vi "Send SMTP.vi"(5 "Attachment file path name":path, 6 "Body":string, 7 "Subject":string, 8 "error in (no error)":errorcluster, 9 "to":string, 10 "from":string, 11 "mail host":string="mailhost.btw-inc.com") -> (0 "error out":errorcluster)   [LabVIEW 2013]
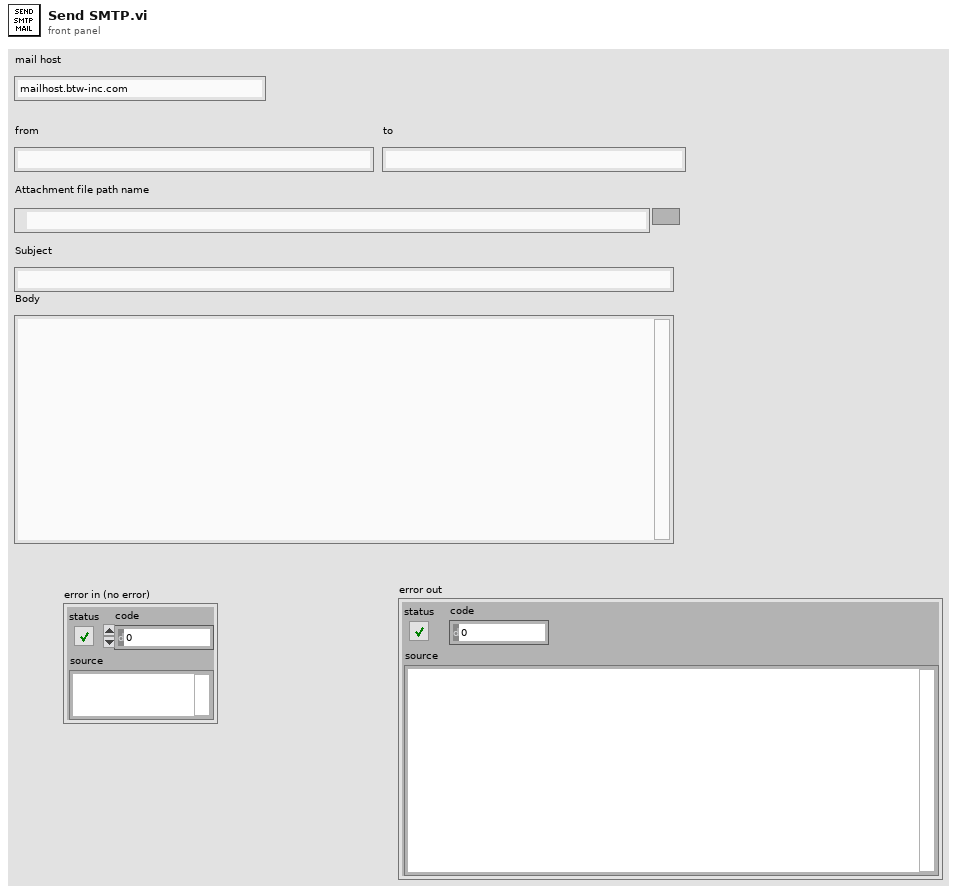
[diagram p1: front panel]
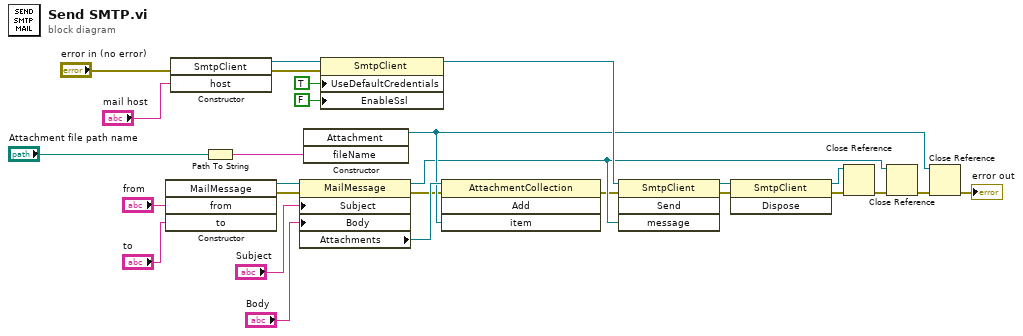
[diagram p0: block diagram]
diagram:
  n1 = constructor class="MailMessage"("from"="from", "to"="to") -> (reference out=w27:refnum<k24>, error out=w26:errorcluster)  [unwired: 3 in, 3 out]
  n2 = constructor class="SmtpClient"(error in="error in (no error)", "host"="mail host") -> (reference out=w25:refnum<k24>, error out=w24:errorcluster)  [unwired: 2 in, 2 out]
  n3 = Path To String(path="Attachment file path name") -> (string=w14:string)
  n4 = property class="MailMessage"(reference=w27, error in=w26, "Subject"="Subject", "Body"="Body") -> (reference out=w3:refnum<k24>, error out=w2:errorcluster, "Attachments"=w12:refnum<k24>)
  n5 = constructor class="Attachment"("fileName"=w14) -> (reference out=w4:refnum<k24>)  [unwired: 3 in, 3 out]
  n6 = property class="SmtpClient"(reference=w25, error in=w24, "UseDefaultCredentials"=TRUE, "EnableSsl"=FALSE ("UseDefaultCredentials")) -> (reference out=w22:refnum<k24>)  [unwired: 1 out]
  n7 = invoke class="AttachmentCollection" method="Add"(reference=w12, error in=w2, "item"=w4) -> (error out=w1:errorcluster)  [unwired: 1 in, 3 out]
  n8 = invoke class="SmtpClient" method="Send"(reference=w22, error in=w1, "message"=w3) -> (reference out=w18:refnum<k24>, error out=w17:errorcluster)  [unwired: 1 in, 2 out]
  n9 = invoke class="SmtpClient" method="Dispose"(reference=w18, error in=w17) -> (reference out=w16:refnum<k24>, error out=w15:errorcluster)  [unwired: 1 in, 1 out]
  n10 = Close Reference(reference=w16, error in (no error)=w15) -> (error out=w21:errorcluster)
  n11 = Close Reference(reference=w3, error in (no error)=w21) -> (error out=w6:errorcluster)
  n12 = Close Reference(reference=w4, error in (no error)=w6) -> (error out=→"error out":errorcluster)
